vi "Get_subDir_Data.vi"(8 "error in (no error)":errorcluster, 11 "AB_Dest_SubDir in":refnum<class "AB_Dest_SubDir.lvclass">) -> (0 "error out":errorcluster, 2 "data":T1, 3 "AB_Dest_SubDir out":refnum<class "AB_Dest_SubDir.lvclass">)   [LabVIEW 2020, in "AB_Dest_SubDir.lvclass"]
uses:
  <vilib>/AppBuilder/AB_Classes/Destination/Dest_SubDirectory/AB_Dest_SubDir.lvclass
  <vilib>/AppBuilder/AB_Classes/Destination/Dest_SubDirectory/AB_SubDirectory.ctl
  <vilib>/AppBuilder/AB_Classes/Destination/Dest_SubDirectory/AB_Dest_SubDir.lvclass/AB_Dest_SubDir.ctl
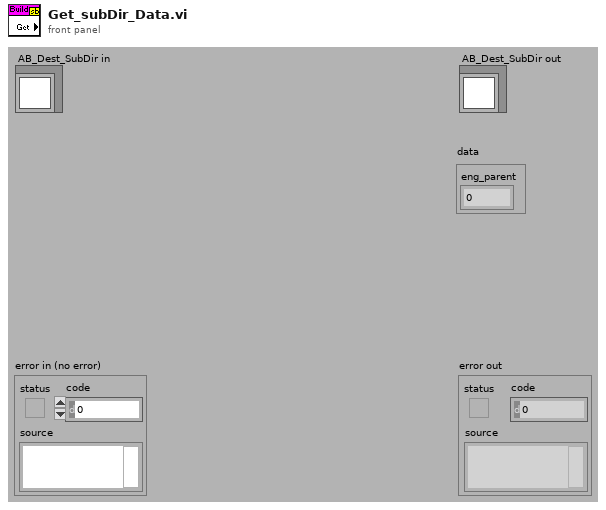
[diagram p1: front panel]
types:
  T1 = typedef "AB_SubDirectory.ctl" = cluster{"eng_parent":i32}
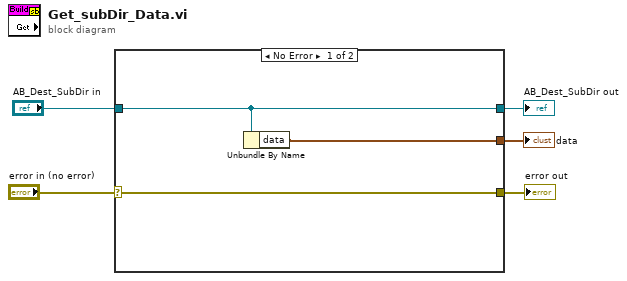
[diagram p0: block diagram]
diagram:
  n1 = case shown="No Error" "error in (no error)" {
    selector: "error in (no error)" -> [w8 w10]
    tunnel: [w8 w10] -> w4
    tunnel: "AB_Dest_SubDir in" -> [w7 w9]
    tunnel: [w7 w9] -> w2
    tunnel: [w6 _] -> w1
    frame No Error {
      n2 = Unbundle By Name(w7) -> ("data"=w6:T1)
    }
    frame Error {
    }
  }
  "error out" <- w4
  "AB_Dest_SubDir out" <- w2
  "data" <- w1
